vi "ColorSense.vi"   [LabVIEW 2016]
uses:
  <vilib>/NXT/Dual Mode Library/Sensors/EV3_Color_RGB.vi
  <vilib>/NXT/Dual Mode Library/Display/drawText.vi
  <vilib>/NXT/NXTIO Xnodes/NXTIONodeSubVIs/LEGOMoveAllMotorsDistance.vi
  <vilib>/NXT/Dual Mode Library/Display/drawNumber.vi
  <vilib>/NXT/Subs/LVHSConnector.ctl
  <vilib>/NXT/NXTIO Xnodes/NXTIOXNode/NXTIO.xnode
  <vilib>/NXT/LegoClasses/BrickReference/BrickReference.lvclass
types:
  T1 = typedef "LVHSConnector.ctl" = refnum<class "BrickReference.lvclass">
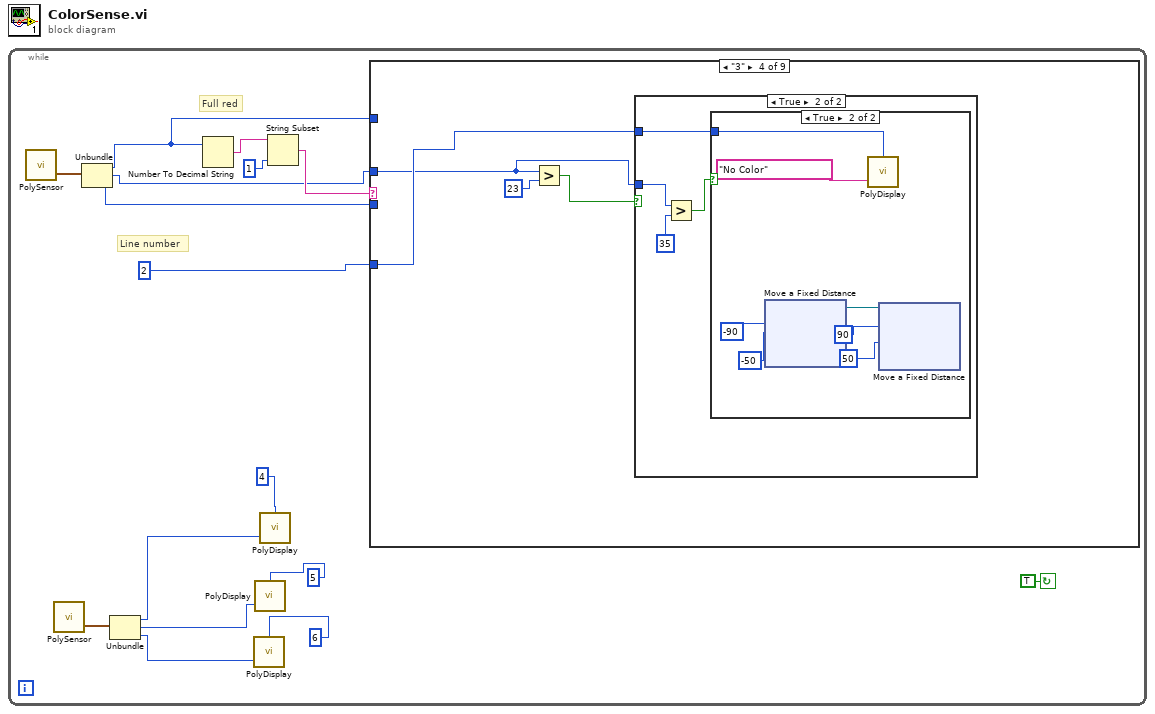
[diagram p0: block diagram]
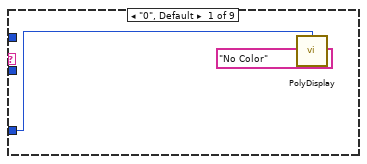
[diagram p2: hidden frame]
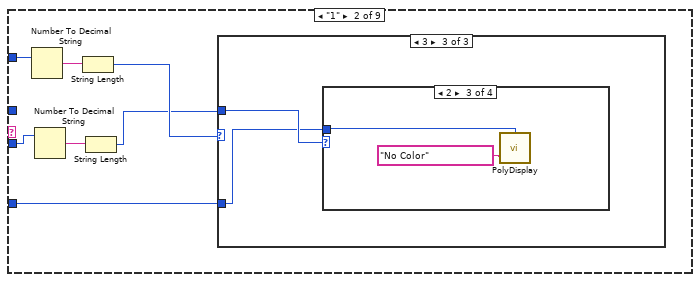
[diagram p3: hidden frame]
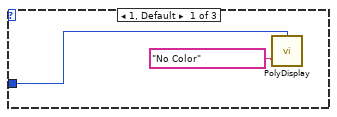
[diagram p4: hidden frame]
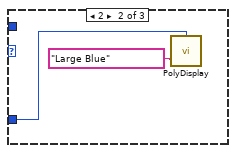
[diagram p5: hidden frame]
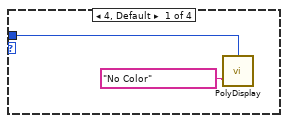
[diagram p6: hidden frame]
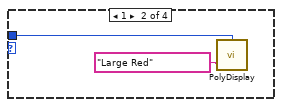
[diagram p7: hidden frame]
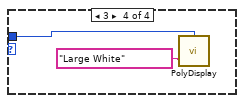
[diagram p8: hidden frame]
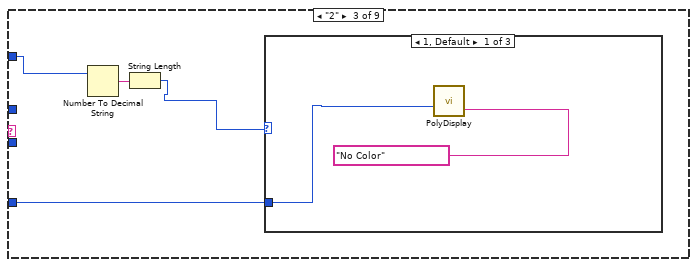
[diagram p9: hidden frame]
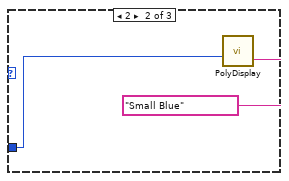
[diagram p10: hidden frame]
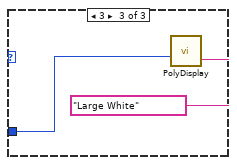
[diagram p11: hidden frame]
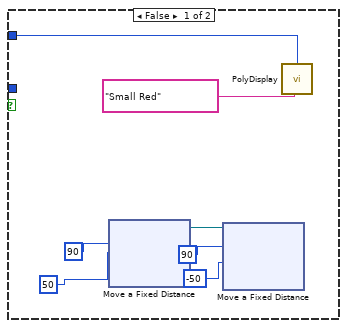
[diagram p12: hidden frame]
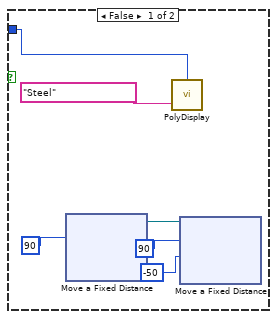
[diagram p13: hidden frame]
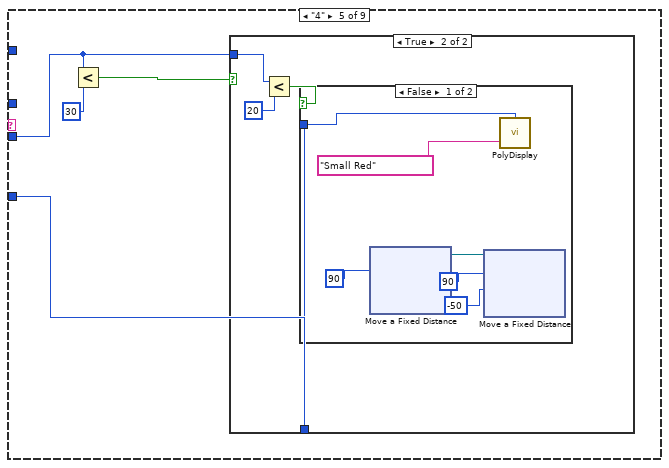
[diagram p14: hidden frame]
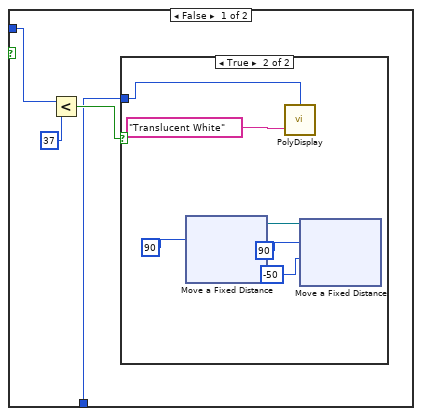
[diagram p15: hidden frame]
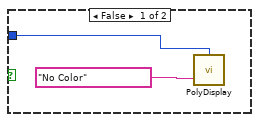
[diagram p16: hidden frame]
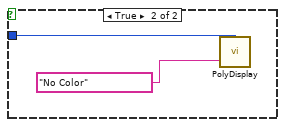
[diagram p17: hidden frame]
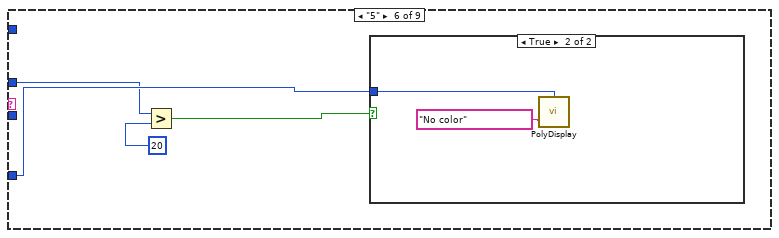
[diagram p18: hidden frame]
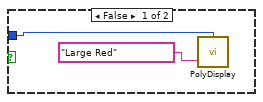
[diagram p19: hidden frame]
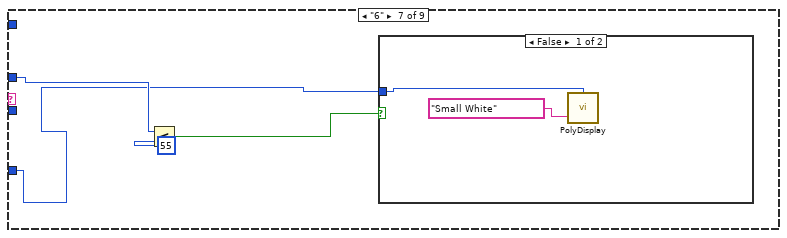
[diagram p20: hidden frame]
diagram:
  n1 = while {
    stop <- TRUE continue-if-true
    # "Full red"
    # "Line number"
    n2 = call-poly <vilib>:"PolySensor.vi"() -> ("RGB Color"=w15:cluster{"Red":u8, "Green":u8, "Blue":u8})  [unwired: 3 in, 1 out]
    n3 = call-poly <vilib>:"PolySensor.vi"() -> ("RGB Color"=w10:cluster{"Red":u8, "Green":u8, "Blue":u8})  [unwired: 3 in, 1 out]
    n4 = Unbundle(w15) -> ("Red"=w11:u8, "Green"=w2:u8, "Blue"=w1:u8)
    n5 = Unbundle(w10) -> ("Red"=w6:u8, "Green"=w5:u8, "Blue"=w4:u8)
    n6 = Number To Decimal String(number=w11) -> (decimal integer string=w14:string)  [unwired: 1 in]
    n7 = call-poly <vilib>:"PolyDisplay.vi"("number"=w4, "Line"=6) -> ()  [unwired: 2 in, 1 out]
    n8 = call-poly <vilib>:"PolyDisplay.vi"("number"=w5, "Line"=5) -> ()  [unwired: 2 in, 1 out]
    n9 = call-poly <vilib>:"PolyDisplay.vi"("number"=w6, "Line"=4) -> ()  [unwired: 2 in, 1 out]
    n10 = String Subset(string=w14, length (rest)=1) -> (substring=w3:string)  [unwired: 1 in]
    n11 = case shown="\"3\"" w3 {
      tunnel: 2 -> [w17 w22 w42 w53 w121 w179 w184 w193 w195]
      tunnel: w11 -> [_ w25 w43 _ _ _ _ _ _]
      tunnel: w2 -> [_ _ _ w50 _ w176 w185 _ _]
      tunnel: w1 -> [_ w21 _ _ w120 _ _ _ _]
      frame "0", Default {
        n12 = call-poly <vilib>:"PolyDisplay.vi"("Text"="No Color", "Line"=w17) -> ()  [unwired: 2 in, 1 out]
      }
      frame "1" {
        n13 = Number To Decimal String(number=w25) -> (decimal integer string=w24:string)  [unwired: 1 in]
        n14 = Number To Decimal String(number=w21) -> (decimal integer string=w20:string)  [unwired: 1 in]
        n15 = String Length(string=w24) -> (length=w23:i32)
        n16 = String Length(string=w20) -> (length=w19:i32)
        n17 = case shown="3" w23 {
          tunnel: w22 -> [w26 w28 w30]
          tunnel: w19 -> [_ _ w31]
          frame 1, Default {
            n18 = call-poly <vilib>:"PolyDisplay.vi"("Text"="No Color", "Line"=w26) -> ()  [unwired: 2 in, 1 out]
          }
          frame 2 {
            n19 = call-poly <vilib>:"PolyDisplay.vi"("Text"="Large Blue", "Line"=w28) -> ()  [unwired: 2 in, 1 out]
          }
          frame 3 {
            n20 = case shown="2" w31 {
              tunnel: w30 -> [w32 w34 w36 w38]
              frame 4, Default {
                n21 = call-poly <vilib>:"PolyDisplay.vi"("Text"="No Color", "Line"=w32) -> ()  [unwired: 2 in, 1 out]
              }
              frame 1 {
                n22 = call-poly <vilib>:"PolyDisplay.vi"("Text"="Large Red", "Line"=w34) -> ()  [unwired: 2 in, 1 out]
              }
              frame 2 {
                n23 = call-poly <vilib>:"PolyDisplay.vi"("Text"="No Color", "Line"=w36) -> ()  [unwired: 2 in, 1 out]
              }
              frame 3 {
                n24 = call-poly <vilib>:"PolyDisplay.vi"("Text"="Large White", "Line"=w38) -> ()  [unwired: 2 in, 1 out]
              }
            }
          }
        }
      }
      frame "2" {
        n25 = Number To Decimal String(number=w43) -> (decimal integer string=w41:string)  [unwired: 1 in]
        n26 = String Length(string=w41) -> (length=w40:i32)
        n27 = case shown="1, Default" w40 {
          tunnel: w42 -> [w44 w46 w48]
          frame 1, Default {
            n28 = call-poly <vilib>:"PolyDisplay.vi"("Text"="No Color", "Line"=w44) -> ()  [unwired: 2 in, 1 out]
          }
          frame 2 {
            n29 = call-poly <vilib>:"PolyDisplay.vi"("Text"="Small Blue", "Line"=w46) -> ()  [unwired: 2 in, 1 out]
          }
          frame 3 {
            n30 = call-poly <vilib>:"PolyDisplay.vi"("Text"="Large White", "Line"=w48) -> ()  [unwired: 2 in, 1 out]
          }
        }
      }
      frame "3" {
        n31 = Greater?(x=w50, y=23) -> (0:w51:bool)
        n32 = case shown="True" w51 {
          tunnel: w53 -> [w59 w78]
          tunnel: w50 -> [_ w76]
          frame False {
            n33 = xnode "Move a Fixed Distance"("Speed 1"=50, "Distance 1"=90) -> ("NXT/EV3"=w56:T1)  [unwired: 2 in]
            n34 = xnode "Move a Fixed Distance"("Speed 1"=-50, "Distance 1"=90, "NXT/EV3"=w56) -> ()  [unwired: 1 in, 1 out]
            n35 = call-poly <vilib>:"PolyDisplay.vi"("Text"="Small Red", "Line"=w59) -> ()  [unwired: 2 in, 1 out]
          }
          frame True {
            n36 = Greater?(x=w76, y=35) -> (0:w75:bool)
            n37 = case shown="True" w75 {
              tunnel: w78 -> [w83 w104]
              frame False {
                n38 = xnode "Move a Fixed Distance"("Distance 1"=90) -> ("NXT/EV3"=w80:T1)  [unwired: 3 in]
                n39 = call-poly <vilib>:"PolyDisplay.vi"("Text"="Steel", "Line"=w83) -> ()  [unwired: 2 in, 1 out]
                n40 = xnode "Move a Fixed Distance"("Speed 1"=-50, "Distance 1"=90, "NXT/EV3"=w80) -> ()  [unwired: 1 in, 1 out]
              }
              frame True {
                n41 = xnode "Move a Fixed Distance"("Speed 1"=-50, "Distance 1"=-90) -> ("NXT/EV3"=w101:T1)  [unwired: 2 in]
                n42 = call-poly <vilib>:"PolyDisplay.vi"("Text"="No Color", "Line"=w104) -> ()  [unwired: 2 in, 1 out]
                n43 = xnode "Move a Fixed Distance"("Speed 1"=50, "Distance 1"=90, "NXT/EV3"=w101) -> ()  [unwired: 1 in, 1 out]
              }
            }
          }
        }
      }
      frame "4" {
        n44 = Less?(x=w120, y=30) -> (x < y?=w123:bool)
        n45 = case shown="True" w123 {
          tunnel: w121 -> [w124 w153]
          tunnel: w120 -> [w126 w151]
          frame False {
            n46 = Less?(x=w126, y=37) -> (x < y?=w125:bool)
            n47 = case shown="True" w125 {
              tunnel: w124 -> [w128 w134]
              frame False {
                n48 = call-poly <vilib>:"PolyDisplay.vi"("Text"="No Color", "Line"=w128) -> ()  [unwired: 2 in, 1 out]
              }
              frame True {
                n49 = xnode "Move a Fixed Distance"("Distance 1"=90) -> ("NXT/EV3"=w131:T1)  [unwired: 3 in]
                n50 = call-poly <vilib>:"PolyDisplay.vi"("Text"="Translucent White", "Line"=w134) -> ()  [unwired: 2 in, 1 out]
                n51 = xnode "Move a Fixed Distance"("Speed 1"=-50, "Distance 1"=90, "NXT/EV3"=w131) -> ()  [unwired: 1 in, 1 out]
              }
            }
          }
          frame True {
            n52 = Less?(x=w151, y=20) -> (x < y?=w150:bool)
            n53 = case shown="False" w150 {
              tunnel: w153 -> [w159 w175]
              frame False {
                n54 = xnode "Move a Fixed Distance"("Distance 1"=90) -> ("NXT/EV3"=w155:T1)  [unwired: 3 in]
                n55 = xnode "Move a Fixed Distance"("Speed 1"=-50, "Distance 1"=90, "NXT/EV3"=w155) -> ()  [unwired: 1 in, 1 out]
                n56 = call-poly <vilib>:"PolyDisplay.vi"("Text"="Small Red", "Line"=w159) -> ()  [unwired: 2 in, 1 out]
              }
              frame True {
                n57 = call-poly <vilib>:"PolyDisplay.vi"("Text"="No Color", "Line"=w175) -> ()  [unwired: 2 in, 1 out]
              }
            }
          }
        }
      }
      frame "5" {
        n58 = Greater?(x=w176, y=20) -> (0:w178:bool)
        n59 = case shown="True" w178 {
          tunnel: w179 -> [w180 w182]
          frame False {
            n60 = call-poly <vilib>:"PolyDisplay.vi"("Text"="Large Red", "Line"=w180) -> ()  [unwired: 2 in, 1 out]
          }
          frame True {
            n61 = call-poly <vilib>:"PolyDisplay.vi"("Text"="No color", "Line"=w182) -> ()  [unwired: 2 in, 1 out]
          }
        }
      }
      frame "6" {
        n62 = Less?(x=w185, y=55) -> (x < y?=w187:bool)
        n63 = case shown="False" w187 {
          tunnel: w184 -> [w188 w190]
          frame False {
            n64 = call-poly <vilib>:"PolyDisplay.vi"("Text"="Small White", "Line"=w188) -> ()  [unwired: 2 in, 1 out]
          }
          frame True {
            n65 = call-poly <vilib>:"PolyDisplay.vi"("Text"="No Color", "Line"=w190) -> ()  [unwired: 2 in, 1 out]
          }
        }
      }
      frame "9" {
        n66 = call-poly <vilib>:"PolyDisplay.vi"("Text"="Large Red", "Line"=w193) -> ()  [unwired: 2 in, 1 out]
      }
      frame "8" {
        n67 = call-poly <vilib>:"PolyDisplay.vi"("Text"="Large Red", "Line"=w195) -> ()  [unwired: 2 in, 1 out]
      }
    }
  }
